vi "TCP Named Service - Client01.vi"() -> ()   [LabVIEW 2016]
doc: "This VI implements a client for the TCP Named Service - Server.vi. It connects to a service by specifying the server address and the name of the service. The client receives the string sent by the server, displays the string and closes the connection."
panel:
  in  "send":bool
  in  "stop":bool
  in  "data in":string="abcdef1234"
  out "Message from Server":string
  # "<AA1300>"
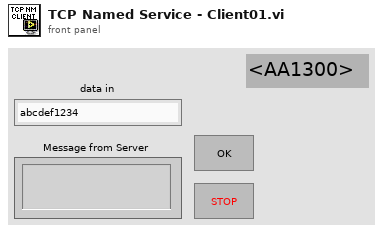
[diagram p1: front panel]
types:
  T1 = enum16{"Standard", "Buffered", "CRLF", "Immediate"}
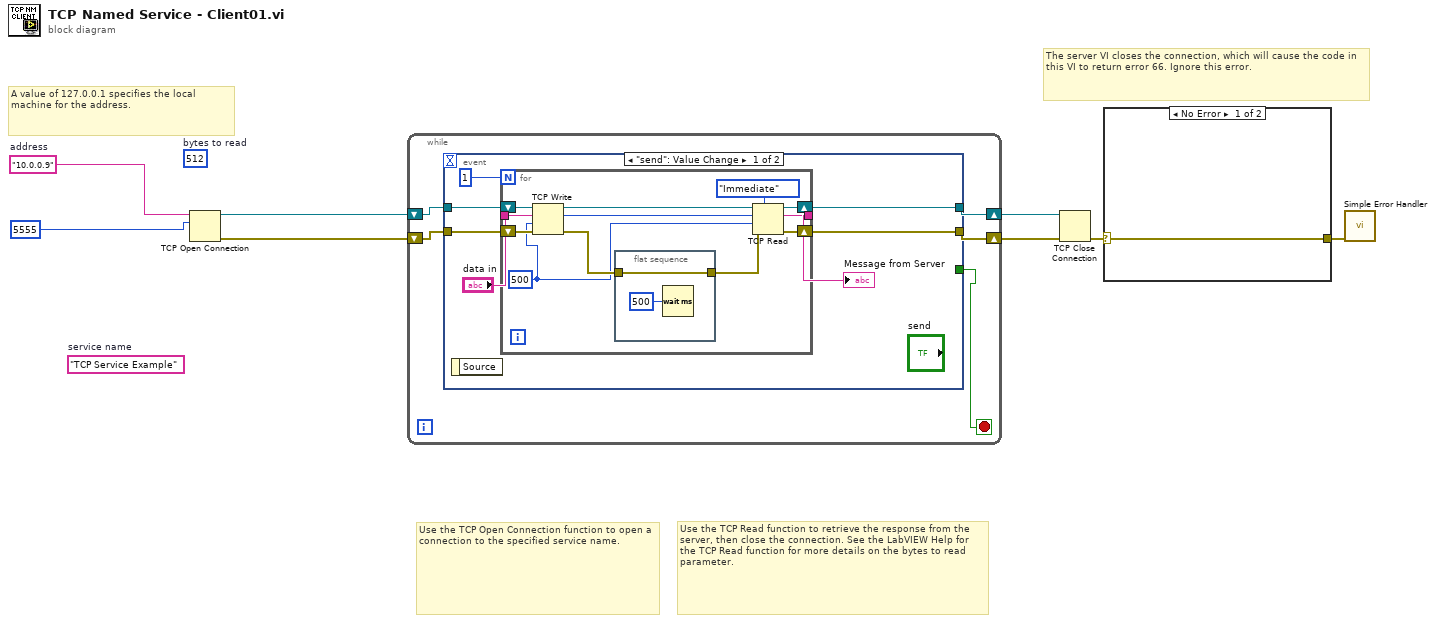
[diagram p0: block diagram]
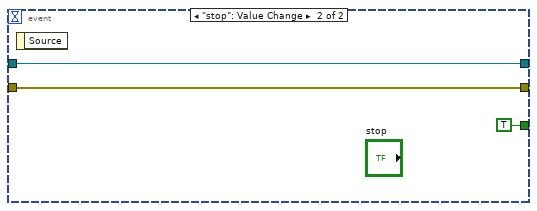
[diagram p2: hidden frame]
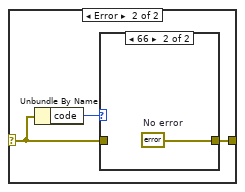
[diagram p3: hidden frame]
diagram:
  (unwired) 512  # bytes to read
  (unwired) "TCP Service Example"  # service name
  w6 = "10.0.0.9"  # address
  # "The server VI closes the connection, which will cause the code in this VI to return error 66. Ignore this error."
  # "A value of 127.0.0.1 specifies the local machine for the address."
  # "Use the TCP Open Connection function to open a connection to the specified service name."
  # "Use the TCP Read function to retrieve the response from the server, then close the connection. See the LabVIEW Help for the TCP Read function for more details on the bytes to read parameter."
  n1 = TCP Open Connection(address=w6, remote port or service name=u16 5555 ("local port (0)")) -> (connection ID=w7:refnum<k5>, error out=w8:errorcluster)  [unwired: 3 in]
  n2 = while {
    shift-right: [w10] -> w1
    shift-left: w8 -> [w13]
    shift-right: [w11] -> w2
    shift-left: w7 -> [w12]
    stop <- w9 stop-if-true
    n3 = event shown="[0] \"send\": Value Change" {
      selector: _ -> [_ _]
      dyn-events: _ -> [_ _]
      timeout: _ -> [_ _]
      tunnel: w13 -> [w20 w35]
      tunnel: w12 -> [w19 w36]
      tunnel: [w18 w36] -> w11
      tunnel: [w17 w35] -> w10
      tunnel: [_ TRUE ("NewVal")] -> w9
      event "send": Value Change {
        n4 = event-data() -> ()  [unwired: 1 in, 1 out]
        n5 = for {
          N: 1 -> [_]
          tunnel: [w28] -> w16
          tunnel: "data in" -> [w24]
          shift-right: [w29] -> w17
          shift-left: w20 -> [w32]
          shift-right: [w30] -> w18
          shift-left: w19 -> [w31]
          w21 = 500 ("timeout ms (25000)")
          n6 = TCP Write(connection ID=w31, data in=w24, error in (no error)=w32, 9:w21) -> (connection ID out=w27:refnum<k5>, bytes written=w22:i32, error out=w26:errorcluster)
          n7 = flat-sequence {
            tunnel: [w33] -> w25
            tunnel: w26 -> [w33]
            frame #0 {
              n8 = Wait (ms)(milliseconds to wait=u32 500) -> ()  [unwired: 1 out]
            }
          }
          n9 = TCP Read(connection ID=w27, bytes to read=w22, error in (no error)=w25, 7:T1."Immediate" ("mode (standard)"), 9:w21) -> (connection ID out=w30:refnum<k5>, data out=w28:string, error out=w29:errorcluster)
        }
        "Message from Server" <- w16
      }
      event "stop": Value Change {
        n10 = event-data() -> ()  [unwired: 1 in, 1 out]
      }
    }
  }
  n11 = TCP Close Connection(connection ID=w2, error in (no error)=w1) -> (error out=w5:errorcluster)  [unwired: 1 in, 1 out]
  n12 = case shown="No Error" w5 {
    selector: w5 -> [w38 w40]
    tunnel: [w38 w39] -> w4
    frame No Error {
    }
    frame Error {
      n13 = Unbundle By Name(w40) -> ("code"=w41:i32)
      n14 = case shown="66" w41 {
        tunnel: w40 -> [w42 _]
        tunnel: [w42 w43] -> w39
        frame Default {
        }
        frame 66 {
          w43 = errorcluster {"status"=FALSE, "code"=0, "source"=""}  # No error
        }
      }
    }
  }
  n15 = call <vilib>:"Simple Error Handler.vi"("error in (no error)"=w4) -> ()  [unwired: 4 in, 5 out]
